vi "StringTag.last_lua.vi"(5 "LuaVIEW reference":T1) -> (15 "error out":errorcluster)   [LabVIEW 2012]
doc: "Returns the last string written to the tag as well as its timestamp. On initialisation, the datalogger rebuffers the last string and its timestamp which is therefore guaranteed to be available without requiring disk I/O.\nParameters:\nobj:strtag\nResults:\nstr:value, last string written to the tag.\nnum:time, timestamp of last written string.\nErrors:\nDead or invalid tag object.\nData logger not initialized."
uses:
  luaview/typedefs/t_LuaVIEW Reference.ctl
  typedefs/t_DataLog Live Tag Strings Methods.ctl
  luaview/subvis/private/LuaVIEW Pull (object).vi
  luaview/subvis/private/LuaVIEW Push (string).vi
  luaview/subvis/private/LuaVIEW Push (number).vi
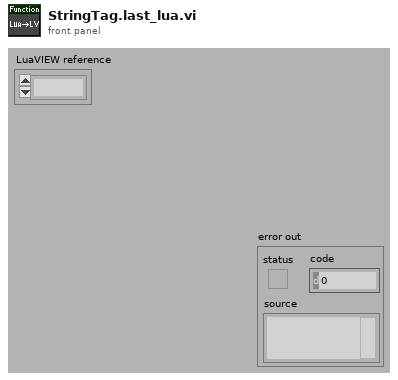
[diagram p1: front panel]
types:
  T1 = typedef "t_LuaVIEW Reference.ctl" = refnum<k1>
  T2 = typedef "t_DataLog Live Tag Strings Methods.ctl" = enum16{"initialize", "rebuffer", "read", "write", "cleanup"}
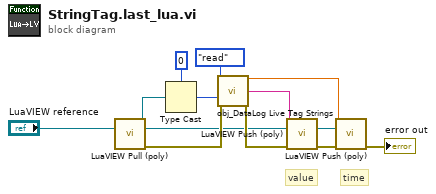
[diagram p0: block diagram]
diagram:
  # "time"
  # "value"
  n1 = call-poly "LuaVIEW Pull (poly).vi"("LuaVIEW reference in"="LuaVIEW reference") -> ("object refnum"=w10:refnum<vi>, "LuaVIEW reference out"=w2:T1, "error out"=w7:errorcluster)  [unwired: 11 in, 1 out]
  n2 = Type Cast(type=0 ("read index in"), x=w10) -> (*(type *) &x=w6:i32)
  n3 = call "obj_DataLog Live Tag Strings.vi"("method"=t_DataLog_Live_Tag_Strings_Methods."read", "tag index"=w6, "error in (no error)"=w7) -> ("time"=w3:dbl, "string out"=w4:string, "error out"=w5:errorcluster)  [unwired: 9 in, 1 out]
  n4 = call-poly "LuaVIEW Push (poly).vi"("string"=w4, "LuaVIEW reference in"=w2, "error in (no error)"=w5) -> ("LuaVIEW reference out"=w13:T1, "error out"=w12:errorcluster)  [unwired: 11 in]
  n5 = call-poly "LuaVIEW Push (poly).vi"("number"=w3, "LuaVIEW reference in"=w13, "error in (no error)"=w12) -> ("error out"=→"error out":errorcluster)  [unwired: 11 in, 1 out]
